vi "Read&WriteFile.vi"   [LabVIEW 2017]
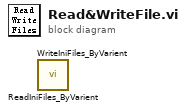
[diagram p0: block diagram]
diagram:
  n1 = call "ReadIniFiles_ByVarient.vi"() -> ()  [unwired: 10 in, 2 out]
  n2 = call "WriteIniFiles_ByVarient.vi"() -> ()  [unwired: 11 in, 1 out]
